vi "BLED1112_auto-connection.vi"(0 "COM Bluegiga in":refnum<visa-resource-name>="COM8", 5 "MAC Address":string="D9:2F:10:92:34:F2", 7 "Address Type":enum16{"Public", "Random"}(ring)=enum."Random") -> (4 "COM out":refnum<visa-resource-name>="COM8", 6 "Connection Ok":bool=TRUE, 8 "Device Name":string="JUN_JUN", 10 "Handle table":string[][](array[string])=[["0001", "1800", "2800"], ["0002", "1800", "2803"], ["0003", "1800", "2A00"], ["0004", "1800", "2803"], ["0005", "1800", "2A01"], ["0006", "1800", "2803"], ["0007", "1800", "2A04"], ["0008", "1801", "2800"], ["0009", "0000F00D1212EFDE1523785FEF13D123", "2800"], ["000A", "0000F00D1212EFDE1523785FEF13D123", "2803"], ["000B", "0000F00D1212EFDE1523785FEF13D123", "000000011212EFDE1523785FEF13D123"], ["000C", "0000F00D1212EFDE1523785FEF13D123", "2902"], ["000D", "000000021212EFDE1523785FEF13D123", "2800"], ["000E", "000000021212EFDE1523785FEF13D123", "2803"], ["000F", "000000021212EFDE1523785FEF13D123", "000000021212EFDE1523785FEF13D123"], ["0010", "000000021212EFDE1523785FEF13D123", "2902"]], 14 "Connection Status":T1={"MAC Address"="D9:2F:10:92:34:F2", "cnx handle"=0, "cnx flags"=5, "Address Type"=1, "Connection Interval (ms)"=15, "Timeout(ms)"=1000, "Latency"=0, "bonding handle"=255} {"Address Type" items=["Public", "Random"]}, 15 "에러 출력":errorcluster={"status"=FALSE, "code"=1073676294, "source"="ble_read_message.vi->ble_read_specific_message.vi->ble_evt_attclient_procedue_completed.vi->ble_write_by_handle_uint8array.vi->ble_write_by_service_characteristic_uint8array.vi->BLED1112_app-connection.vi->[BLE Test] ble_read_write_characteristics.vi 안에 VISA 읽기"})   [LabVIEW 2015]
uses:
  Lib_Bled112 toolkit/type_def/connection_status_bundle.ctl
  Lib_Bled112 toolkit/type_def/address_type.ctl
  Lib_Bled112 toolkit/ble_functions/ble_write_by_handle_uint8array.vi
panel:
  in  "reconnection loop end":bool
  out "Scan success?":bool
  out "BLED112 Dongle Info":string="Major: 1, Minor: 3, Patch: 2, Build: 122, LL ver: 3, Protocol ver: 1 and HW ver: 3  "
  out "Timeout Error":bool
  in  "Timeout":dbl=120.0
  in  "Stop":bool
  out "Message":string
  out "Get Device name?":bool=TRUE
  out "Get handle table?":bool=TRUE
  out "Connected?":bool=TRUE
  # "BLE Connection"
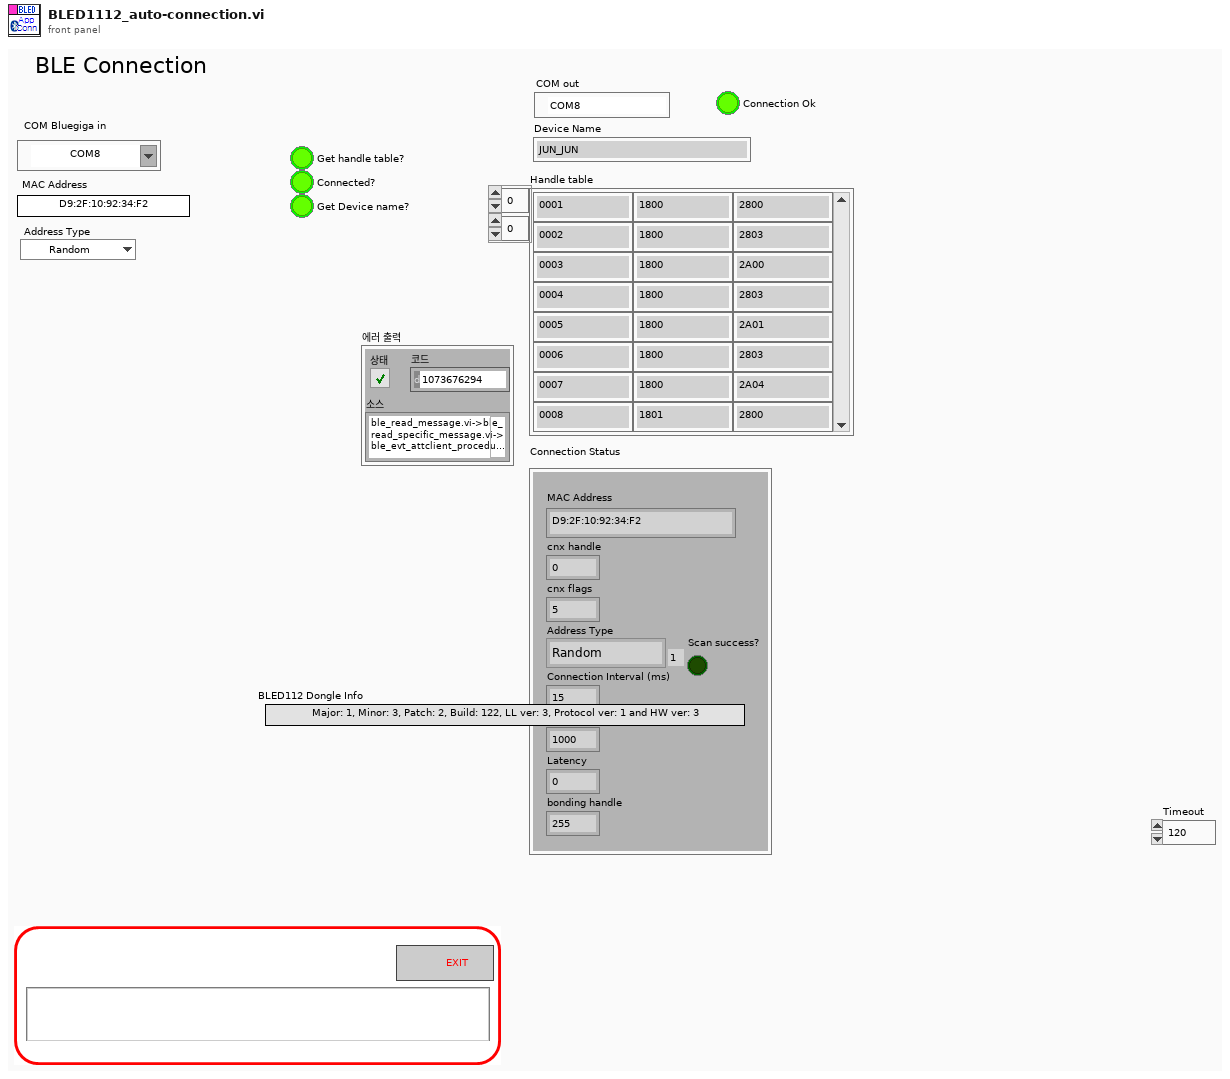
[diagram p1: front panel]
types:
  T1 = typedef "connection_status_bundle.ctl" = cluster{"MAC Address":string, "cnx handle":u8, "cnx flags":u8, "Address Type":T2, "Connection Interval (ms)":u16, "Timeout(ms)":u16, "Latency":u16, "bonding handle":u8}
  T2 = typedef "address_type.ctl" = u8
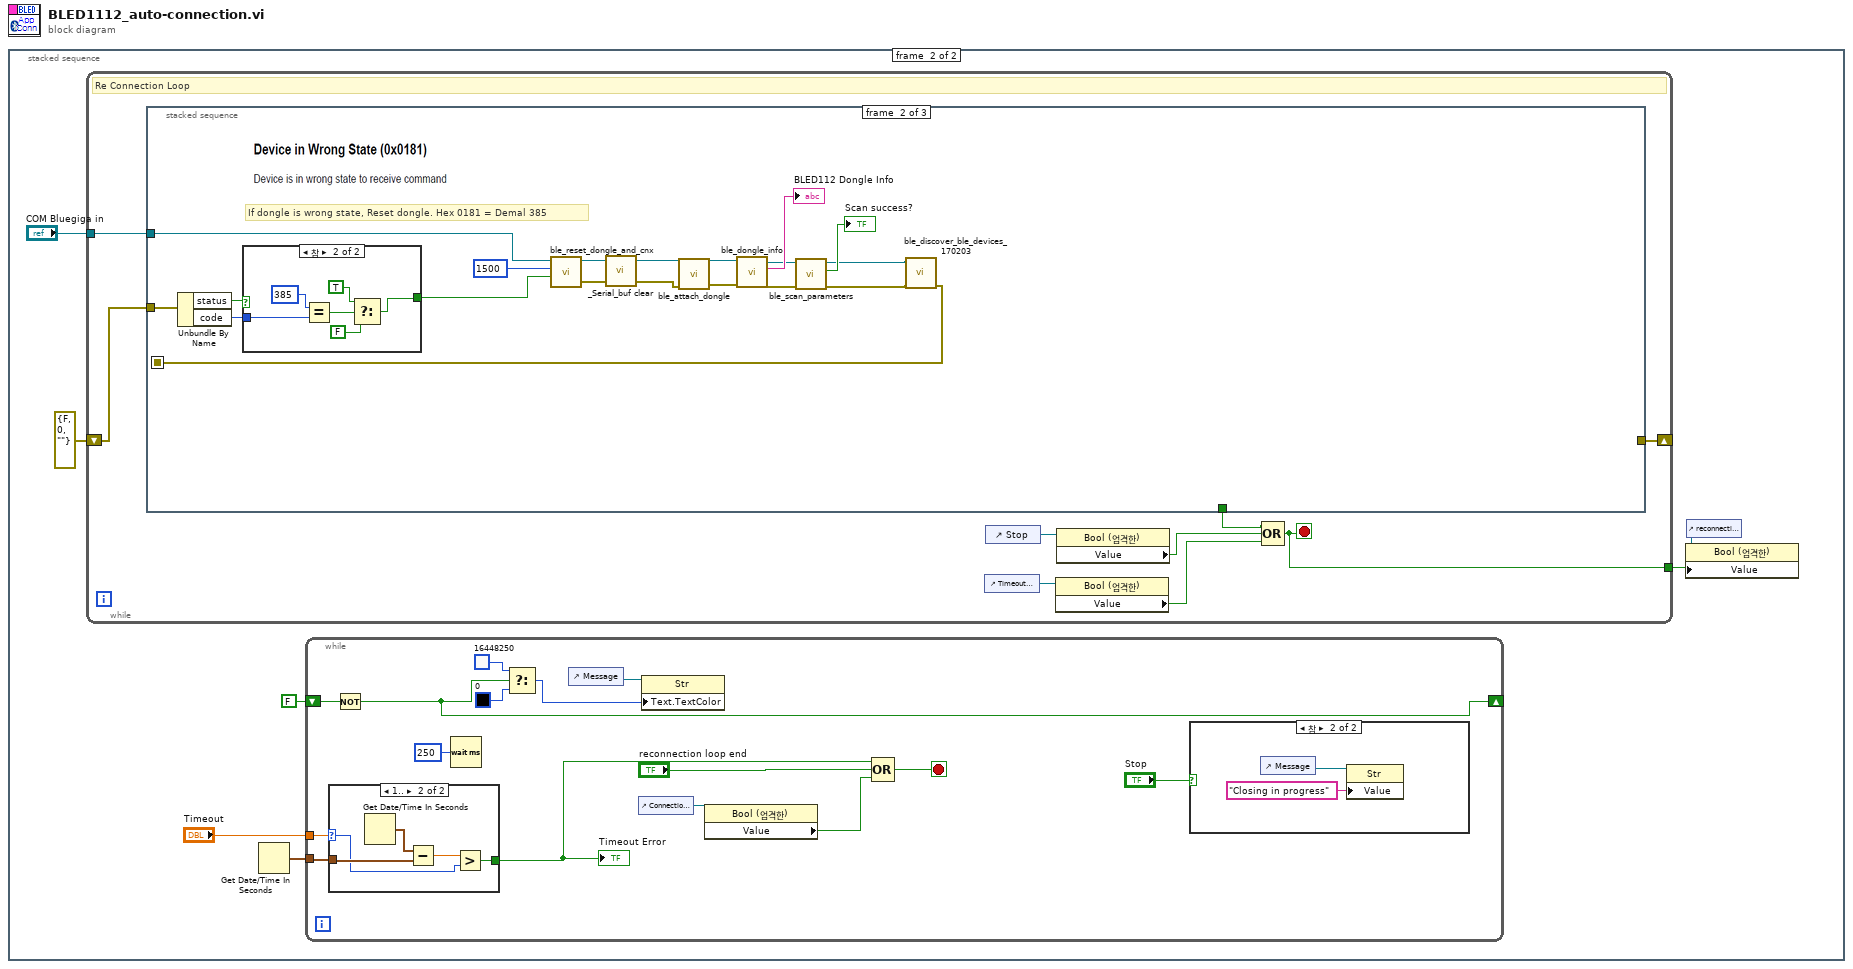
[diagram p0: block diagram]
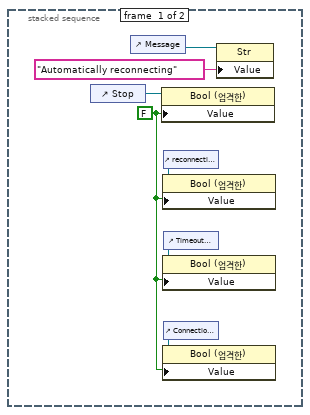
[diagram p2: hidden frame]
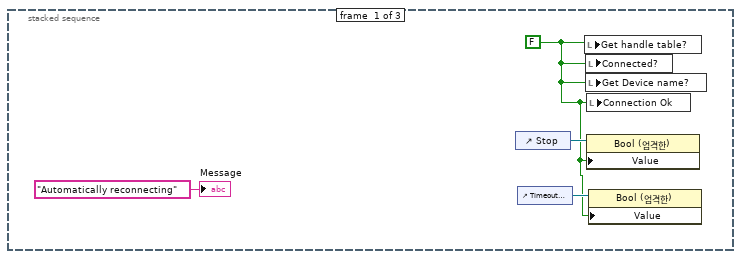
[diagram p3: hidden frame]
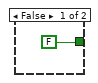
[diagram p4: hidden frame]
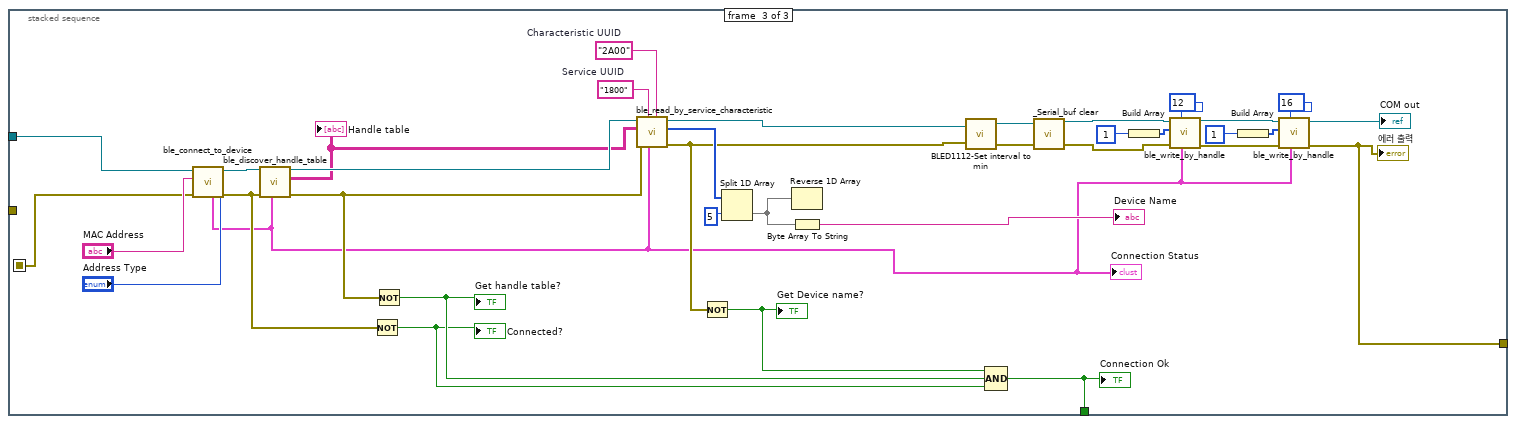
[diagram p5: hidden frame]
diagram:
  n1 = stacked-sequence {
    frame #0 {
      w1 = FALSE ("값")
      n2 = control-ref of="Stop"() -> (w5:refnum<vi>)
      n3 = control-ref of="Message"() -> (w6:refnum<vi>)
      n4 = property class="Bool (엄격한)"(reference=w5, "Value"=w1) -> ()  [unwired: 1 in, 2 out]
      n5 = control-ref of="reconnection loop end"() -> (w4:refnum<vi>)
      n6 = property class="Bool (엄격한)"(reference=w4, "Value"=w1) -> ()  [unwired: 1 in, 2 out]
      n7 = control-ref of="Timeout Error"() -> (w3:refnum<vi>)
      n8 = property class="Bool (엄격한)"(reference=w3, "Value"=w1) -> ()  [unwired: 1 in, 2 out]
      n9 = control-ref of="Connection Ok"() -> (w2:refnum<vi>)
      n10 = property class="Bool (엄격한)"(reference=w2, "Value"=w1) -> ()  [unwired: 1 in, 2 out]
      n11 = property class="Str"(reference=w6, "Value"="Automatically reconnecting" ("값")) -> ()  [unwired: 1 in, 2 out]
    }
    frame #1 {
      n12 = while {
        tunnel: "COM Bluegiga in" -> [w18]
        tunnel: [w17] -> w9
        shift-right: [w16] -> _
        shift-left: errorcluster {"status"=FALSE, "code"=0, "source"=""} ("에러 상수") -> [w15]
        stop <- w17 stop-if-true
        # "Re Connection Loop"
        n13 = stacked-sequence {
          seq-local: [_ w45 _] -> [_ _ w67]
          tunnel: [_ _ w89] -> w22
          tunnel: w18 -> [_ w46 w68]
          tunnel: [_ _ w54] -> w16
          tunnel: w15 -> [_ w31 _]
          frame #0 {
            w24 = FALSE ("Get handle table?")
            n14 = control-ref of="Stop"() -> (w26:refnum<vi>)
            n15 = control-ref of="Timeout Error"() -> (w25:refnum<vi>)
            n16 = local write "Get handle table?"(w24) -> ()
            n17 = local write "Connected?"(w24) -> ()
            n18 = local write "Get Device name?"(w24) -> ()
            n19 = local write "Connection Ok"(w24) -> ()
            n20 = property class="Bool (엄격한)"(reference=w26, "Value"=w24) -> ()  [unwired: 1 in, 2 out]
            n21 = property class="Bool (엄격한)"(reference=w25, "Value"=w24) -> ()  [unwired: 1 in, 2 out]
            "Message" <- "Automatically reconnecting" ("Message")
          }
          frame #1 {
            # "If dongle is wrong state, Reset dongle. Hex 0181 = Demal 385"
            n22 = Unbundle By Name(w31) -> ("status"=w30:bool, "code"=w29:i32)
            n23 = case shown="참" w30 {
              tunnel: w29 -> [_ w53]
              tunnel: [FALSE ("Reset?") w48] -> w28
              frame False {
              }
              frame True {
                n24 = Equal?(x=385 ("wait time (100)"), y=w53) -> (x = y?=w51:bool)
                n25 = Select(t=TRUE ("Reset?"), s=w51, f=FALSE ("Reset?")) -> (s? t:f=w48:bool)
              }
            }
            n26 = call "ble_reset_dongle_and_cnx.vi"("Reset?"=w28, "wait time (100)"=u32 1500, "COM Bluegiga in"=w46) -> ("error out"=w37:errorcluster, "COM Bluegiga out"=w38:refnum<visa-resource-name>)  [unwired: 7 in]
            n27 = call "_Serial_buf clear.vi"("에러 출력 2"=w37, "Serial Port"=w38) -> ("에러 출력"=w35:errorcluster, "Serial Port 2"=w36:refnum<visa-resource-name>)  [unwired: 2 in]
            n28 = call "ble_attach_dongle.vi"("error in (no error)"=w35, "COM Bluegiga in"=w36) -> ("error out"=w40:errorcluster, "COM Bluegiga out"=w41:refnum<visa-resource-name>)  [unwired: 8 in]
            n29 = call "ble_dongle_info.vi"("error in (no error)"=w40, "COM Bluegiga in"=w41) -> ("error out"=w42:errorcluster, "info"=→"BLED112 Dongle Info":string, "COM Bluegiga out"=w43:refnum<visa-resource-name>)  [unwired: 7 in]
            n30 = call "ble_scan_parameters.vi"("error in (no error)"=w42, "COM Bluegiga in"=w43) -> ("error out"=w33:errorcluster, "success?"=→"Scan success?":bool, "COM Bluegiga out"=w32:refnum<visa-resource-name>)  [unwired: 7 in]
            n31 = call "ble_discover_ble_devices_170203.vi"("error in (no error)"=w33, "COM Bluegiga in"=w32) -> ("error out"=w45:errorcluster)  [unwired: 7 in, 2 out]
          }
          frame #2 {
            w84 = "2A00"  # Characteristic UUID
            w85 = "1800"  # Service UUID
            n32 = call "ble_connect_to_device.vi"("Address Type"="Address Type", "error in (no error)"=w67, "MAC Address"="MAC Address", "COM Bluegiga in"=w68) -> ("error out"=w80:errorcluster, "COM Bluegiga out"=w81:refnum<visa-resource-name>, "Connection Status"=w56:T1)  [unwired: 5 in]
            "Connection Status" <- w56
            n33 = call "ble_discover_handle_table.vi"("Connection Status"=w56, "error in (no error)"=w80, "COM Bluegiga in"=w81) -> ("error out"=w79:errorcluster, "Handle table"=w69:string[][], "COM Bluegiga out"=w88:refnum<visa-resource-name>)  [unwired: 6 in]
            "Handle table" <- w69
            n34 = Not(x=w80) -> (.not. x?=w70:bool)
            "Connected?" <- w70
            n35 = Not(x=w79) -> (.not. x?=w71:bool)
            "Get handle table?" <- w71
            n36 = call "ble_read_by_service_characteristic.vi"("Characteristic UUID"=w84, "Connection Status"=w56, "Service UUID"=w85, "error in (no error)"=w79, "Handle table"=w69, "COM Bluegiga in"=w88) -> ("error out"=w77:errorcluster, "characteristic value"=w83:u8[], "COM Bluegiga out"=w78:refnum<visa-resource-name>)  [unwired: 3 in]
            n37 = Not(x=w77) -> (.not. x?=w72:bool)
            "Get Device name?" <- w72
            n38 = Split 1D Array(array=w83, index=5) -> (second subarray=w82:u8[])  [unwired: 1 out]
            n39 = Reverse 1D Array(array=w82) -> ()  [unwired: 1 out]
            n40 = Byte Array To String(unsigned byte array=w82) -> (string=→"Device Name":string)
            n41 = call "BLED1112-Set interval to min.vi"("에러 입력(에러 없음)"=w77, "VISA 리소스 이름"=w78) -> ("에러 출력"=w75:errorcluster, "VISA 리소스 이름 출력"=w76:refnum<visa-resource-name>)
            n42 = Compound Arithmetic op=AND ("복합 연산")(w72, w71, w70) -> (w89:bool)
            "Connection Ok" <- w89
            n43 = call "_Serial_buf clear.vi"("에러 출력 2"=w75, "Serial Port"=w76) -> ("에러 출력"=w62:errorcluster, "Serial Port 2"=w63:refnum<visa-resource-name>)  [unwired: 2 in]
            n44 = Build Array(u16 1 ("Handle")) -> (w66:u16[])
            n45 = call-poly "ble_write_by_handle.vi"("Connection Status"=w56, "Handle"=u16 12, "error in (no error)"=w62, "data (uint8array)"=w66, "COM Bluegiga in"=w63) -> ("error out"=w57:errorcluster, "COM Bluegiga out"=w58:refnum<visa-resource-name>)  [unwired: 5 in]
            n46 = Build Array(u16 1 ("Handle")) -> (w59:u16[])
            n47 = call-poly "ble_write_by_handle.vi"("Connection Status"=w56, "Handle"=u16 16, "error in (no error)"=w57, "data (uint8array)"=w59, "COM Bluegiga in"=w58) -> ("error out"=w54:errorcluster, "COM Bluegiga out"=→"COM out":refnum<visa-resource-name>)  [unwired: 5 in]
            "에러 출력" <- w54
          }
        }
        n48 = control-ref of="Timeout Error"() -> (w23:refnum<vi>)
        n49 = control-ref of="Stop"() -> (w21:refnum<vi>)
        n50 = property class="Bool (엄격한)"(reference=w23) -> ("Value"=w19:bool)  [unwired: 1 in, 2 out]
        n51 = property class="Bool (엄격한)"(reference=w21) -> ("Value"=w20:bool)  [unwired: 1 in, 2 out]
        n52 = Compound Arithmetic op=OR ("복합 연산")(w22, w20, w19) -> (w17:bool)
      }
      n53 = Get Date/Time In Seconds() -> (seconds since 1Jan1904=w13:timestamp)
      n54 = while {
        shift-right: [w93] -> _
        shift-left: FALSE -> [w103]
        tunnel: w13 -> [w101]
        tunnel: "Timeout" -> [w100]
        stop <- w98 stop-if-true
        n55 = case shown="1.." w100 {
          selector: w100 -> [_ w108]
          tunnel: w101 -> [_ w110]
          tunnel: [_ w107] -> w99
          frame 0, Default {
          }
          frame 1.. {
            n56 = Get Date/Time In Seconds() -> (seconds since 1Jan1904=w111:timestamp)
            n57 = Subtract(x=w111, y=w110) -> (x-y=w109:dbl)
            n58 = Greater?(x=w109, y=w108) -> (0:w107:bool)
          }
        }
        "Timeout Error" <- w99
        n59 = Not(x=w103) -> (.not. x?=w93:bool)
        n60 = Wait (ms)(milliseconds to wait=u32 250 ("대기 시간(ms)")) -> ()  [unwired: 1 out]
        n61 = Select(t=u32 16448250, s=w93, f=u32 0) -> (s? t:f=w90:u32)
        n62 = control-ref of="Message"() -> (w104:refnum<vi>)
        n63 = control-ref of="Connection Ok"() -> (w97:refnum<vi>)
        n64 = property class="Str"(reference=w104, "Text.TextColor"=w90) -> ()  [unwired: 1 in, 2 out]
        n65 = property class="Bool (엄격한)"(reference=w97) -> ("Value"=w96:bool)  [unwired: 1 in, 2 out]
        n66 = Compound Arithmetic op=OR ("복합 연산")(w99, "reconnection loop end", w96) -> (w98:bool)
        n67 = case shown="참" "Stop" {
          frame False {
          }
          frame True {
            n68 = control-ref of="Message"() -> (w106:refnum<vi>)
            n69 = property class="Str"(reference=w106, "Value"="Closing in progress" ("값")) -> ()  [unwired: 1 in, 2 out]
          }
        }
      }
      n70 = control-ref of="reconnection loop end"() -> (w10:refnum<vi>)
      n71 = property class="Bool (엄격한)"(reference=w10, "Value"=w9) -> ()  [unwired: 1 in, 2 out]
    }
  }
